vi "Read Var Info.vi"(0 "SharedVariableWrapper in":refnum<class "SharedVariableWrapper.lvclass">, 5 "name":string, 11 "error in":errorcluster) -> (6 "key not found?":bool, 8 "need to update?":bool, 10 "value":T1, 15 "error out":errorcluster)   [LabVIEW 2019, in "SharedVariableWrapper.lvclass"]
uses:
  SharedVariableWrapper.lvclass
  shared variable info.ctl
  SharedVariableWrapper.lvclass/SharedVariableWrapper.ctl
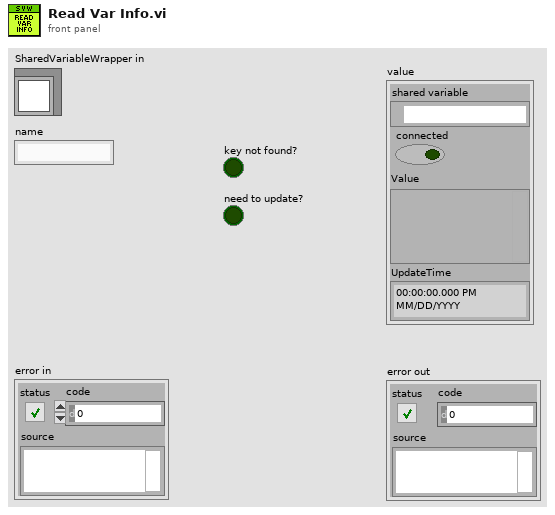
[diagram p1: front panel]
types:
  T1 = typedef "SharedVariableWrapper.lvclass/shared variable info.ctl" = cluster{"shared variable":refnum<k21>, "connected":bool, "Value":variant, "UpdateTime":timestamp}
  T2 = typedef "SharedVariableWrapper.lvclass/Config.ctl" = cluster{"connection str":string, "timeout":dbl, "ip":string}
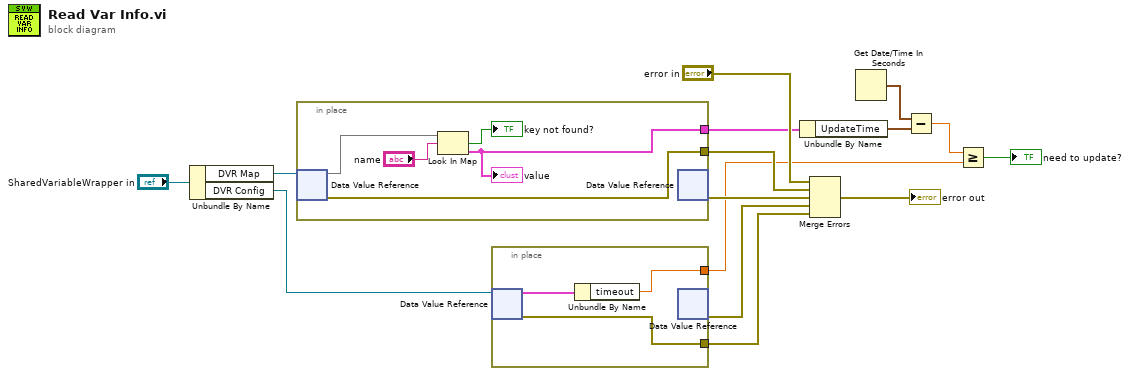
[diagram p0: block diagram]
diagram:
  n1 = Unbundle By Name("SharedVariableWrapper in") -> ("DVR Map"=w14:refnum<data-value>, "DVR Config"=w9:refnum<data-value>)
  n2 = in-place {
    in-place-border: [w20] -> w8
    in-place-border: [w18] -> w11
    n3 = in-place-dvr #1(w14) -> (w19:map{string, T1}, w18:errorcluster)
    n4 = Look In Map(map=w19, key="name") -> (key not found?=→"key not found?":bool, value=w20:T1)  [unwired: 1 in]
    "value" <- w20
    n5 = in-place-dvr #1() -> (w10:errorcluster)  [unwired: 1 in, 1 out]
  }
  n6 = in-place {
    in-place-border: [w23] -> w1
    in-place-border: [w21] -> w4
    n7 = in-place-dvr #2(w9) -> (w22:T2, w23:errorcluster)
    n8 = Unbundle By Name(w22) -> ("timeout"=w21:dbl)
    n9 = in-place-dvr #2() -> (w2:errorcluster)  [unwired: 1 in, 1 out]
  }
  n10 = Unbundle By Name(w8) -> ("UpdateTime"=w7:timestamp)
  n11 = Merge Errors("error in", w11, w10, w2, w1) -> (→"error out":errorcluster)
  n12 = Get Date/Time In Seconds() -> (seconds since 1Jan1904=w6:timestamp)
  n13 = Subtract(x=w6, y=w7) -> (x-y=w5:dbl)
  n14 = Greater Or Equal?(x=w5, y=w4) -> (x >= y?=→"need to update?":bool)
